vi "Main (Blick).vi"() -> ()   [LabVIEW 2018]
uses:
  <vilib>/platform/TimedLoop/XDataNode/XDataNode.xnode
  <vilib>/Platform/TimedLoop/XDataNode/nitl_modes.ctl
  <vilib>/Platform/TimedLoop/XDataNode/XDNodeRunTimeDep.lvlib
  <vilib>/Platform/TimedLoop/XDataNode/wakeup.ctl
  <vilib>/Platform/TimedLoop/XDataNode/timing_clust.ctl
  <extravilib>/ChannelInstances/Tag-bool.lvlib
panel:
  out "1 3":bool
  out "1 2":bool
  out "1":bool
  in  "OK Button":bool
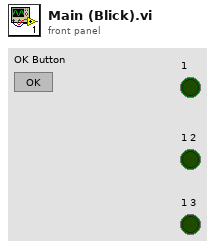
[diagram p1: front panel]
types:
  T1 = typedef "XDNodeRunTimeDep.lvlib/timing_clust.ctl" = cluster{"Expected End [f-1]":u64, "Actual End [f-1]":u64, "Finished Late? [f-1]":bool, "Expected End [i-1]":u64, "Actual End [i-1]":u64, "Finished Late? [i-1]":bool, "Expected Start [i]":u64, "Actual Start [i]":u64, "Expected Start [f]":u64, "Actual Start [f]":u64, "Source Name":string, "Structure Name":string, "Period":i64, "Deadline":i64, "Offset":i64, "Start":i64, "Priority":i32, "Timeout":i32, "Mode":T2, "Wakeup Reason":T3, "Error":errorcluster, "Source Type":string, "Secondary Source Type":string, "Global End Time":u64, "Global Start Time":u64, "Frame Duration":u64, "Iteration Duration":u64, "Assigned CPU":i32, "I/O Scan Engine Mode":u32}
  T2 = typedef "XDNodeRunTimeDep.lvlib/nitl_modes.ctl" = enum32{"No Change", "Process missed periods, maintain original phase", "Discard missed periods, maintain original phase", "Process missed periods, ignore original phase", "Discard missed periods, ignore original phase"}
  T3 = typedef "XDNodeRunTimeDep.lvlib/wakeup.ctl" = enum32{"Normal", "Aborted", "Asynchronous wakeup", "Timing source error", "Timed loop error", "Timeout"}
  T4 = typedef "Tag-bool.lvlib/))Channel.ctl" = refnum<queue>
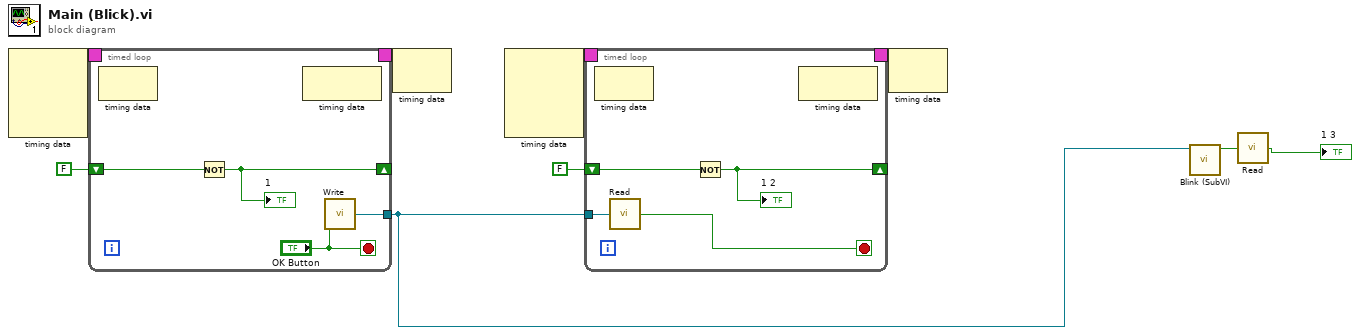
[diagram p0: block diagram]
diagram:
  n1 = node-c288() -> (w9:T1)  [unwired: 4 in]
  n2 = timed-loop {
    timing: w9 -> [_]
    timing-out: [_] -> w8
    shift-right: [w12] -> _
    shift-left: FALSE -> [w13]
    tunnel: [w10] -> w3
    stop <- "OK Button" stop-if-true
    n3 = node-c288() -> ()  [unwired: 1 in, 1 out]
    n4 = Not(x=w13) -> (.not. x?=w12:bool)
    "1" <- w12
    n5 = node-c288() -> ()  [unwired: 1 in, 1 out]
    n6 = call <extravilib>:"Write.vi"("element"="OK Button") -> ("channel"=w10:T4)  [unwired: 1 out]
  }
  n7 = node-c288(w8) -> ()  [unwired: 1 out]
  n8 = node-c288() -> (w6:T1)  [unwired: 4 in]
  n9 = timed-loop {
    timing: w6 -> [_]
    timing-out: [_] -> w5
    shift-right: [w18] -> _
    shift-left: FALSE -> [w19]
    tunnel: w3 -> [w17]
    stop <- w16 stop-if-true
    n10 = node-c288() -> ()  [unwired: 1 in, 1 out]
    n11 = call <extravilib>:"Read.vi"("channel"=w17) -> ("element"=w16:bool)  [unwired: 1 in, 1 out]
    n12 = Not(x=w19) -> (.not. x?=w18:bool)
    "1 2" <- w18
    n13 = node-c288() -> ()  [unwired: 1 in, 1 out]
  }
  n14 = node-c288(w5) -> ()  [unwired: 1 out]
  n15 = call "Blink (SubVI).vi"("Channel in"=w3) -> ("1 3"=w2:bool)  [unwired: 10 in]
  n16 = call <extravilib>:"Read.vi"("channel"=w2) -> ("element"=→"1 3":bool)  [unwired: 1 in, 1 out]
